vi "Configure Probe (Channel).vi"(6 "Operation (0: Setup)":i32(ring) items=["Setup", "Auto Zero", "Degauss"], 7 "Input Mode (1: Pass)":i32(ring)=1 items=["Bypass", "Pass"], 8 "error in (no error)":errorcluster, 9 "Forced Range (0)":dbl, 10 "Channel (0: Channel 1)":i32(ring) items=["Channel 1", "Channel 2", "Channel 3", "Channel 4"], 11 "VISA resource name":refnum<visa-resource-name>) -> (0 "error out":errorcluster, 3 "VISA resource name out":refnum<visa-resource-name>)   [LabVIEW 2009, in "Tektronix DPO MSO 2000 4000 Series.lvlib"]
doc: "Configures settings of a probe attached to the specified channel for an oscilloscope."
uses:
  <instrlib>/Tektronix DPO MSO 2000 4000 Series/Tektronix DPO MSO 2000 4000 Series.lvlib
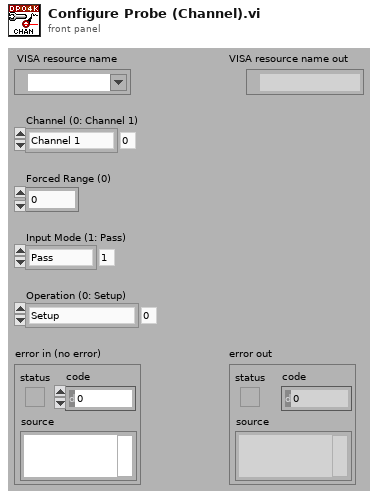
[diagram p1: front panel]
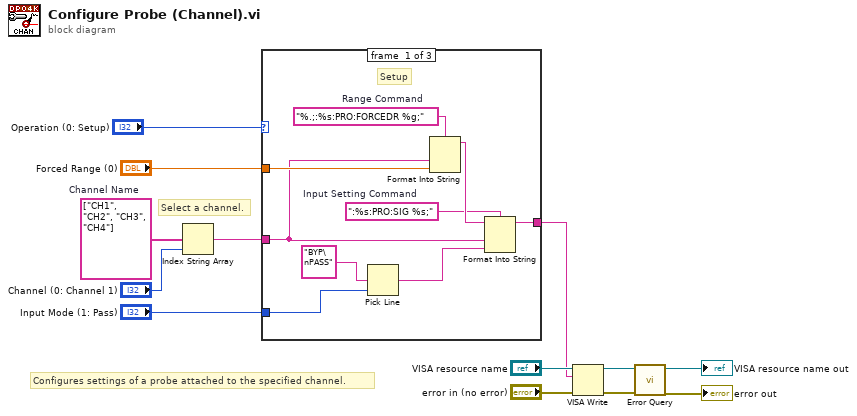
[diagram p0: block diagram]
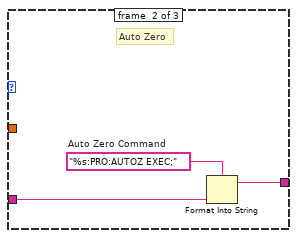
[diagram p2: hidden frame]
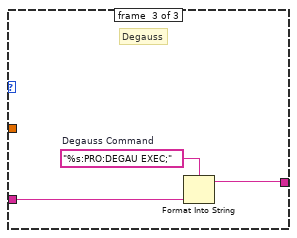
[diagram p3: hidden frame]
diagram:
  w6 = string[] ["CH1", "CH2", "CH3", "CH4"]  # Channel Name
  # "Select a channel."
  # "Configures settings of a probe attached to the specified channel."
  n1 = Index String Array(1:"Channel (0: Channel 1)", 2:w6) -> (0:w4:string)  [unwired: 1 in]
  n2 = case shown="0, Default" "Operation (0: Setup)" {
    tunnel: "Forced Range (0)" -> [w22 _ _]
    tunnel: [w20 w24 w27] -> w2
    tunnel: w4 -> [w19 w23 w26]
    tunnel: "Input Mode (1: Pass)" -> [w14 _ _]
    frame #0 {
      w17 = ":%s:PRO:SIG %s;"  # Input Setting Command
      w18 = "%.;:%s:PRO:FORCEDR %g;"  # Range Command
      # "Setup"
      n3 = Pick Line(multi-line string="BYP\nPASS", line index=w14) -> (output string=w15:string)  [unwired: 1 in]
      n4 = Format Into String(format string=w18, w19, w22) -> (resulting string=w21:string)  [unwired: 2 in, 1 out]
      n5 = Format Into String(format string=w17, initial string=w21, w19, w15) -> (resulting string=w20:string)  [unwired: 1 in, 1 out]
    }
    frame #1 {
      w25 = "%s:PRO:AUTOZ EXEC;"  # Auto Zero Command
      # "Auto Zero"
      n6 = Format Into String(format string=w25, w23) -> (resulting string=w24:string)  [unwired: 2 in, 1 out]
    }
    frame #2 {
      w28 = "%s:PRO:DEGAU EXEC;"  # Degauss Command
      # "Degauss"
      n7 = Format Into String(format string=w28, w26) -> (resulting string=w27:string)  [unwired: 2 in, 1 out]
    }
  }
  n8 = VISA Write(VISA resource name="VISA resource name", write buffer=w2, error in (no error)="error in (no error)") -> (VISA resource name out=w11:refnum<visa-resource-name>, error out=w10:errorcluster)  [unwired: 1 out]
  n9 = call <instrlib>:"Error Query.vi"("error in (no error)"=w10, "VISA resource name"=w11) -> ("error out"=→"error out":errorcluster, "VISA resource name out"=→"VISA resource name out":refnum<visa-resource-name>)  [unwired: 6 in, 2 out]
